vi "Unloading_Queue_States.vi"(7 "QUEUE ST":T2=enum."CLOSE Q", 8 "error in":errorcluster, 11 "Unload St":T1[](array[typedef])) -> (0 "error OUT":errorcluster, 3 "Unload ST":T1)   [LabVIEW 2017]
uses:
  Controls/QUEUE_STATES.ctl
  Controls/Unload_St.ctl
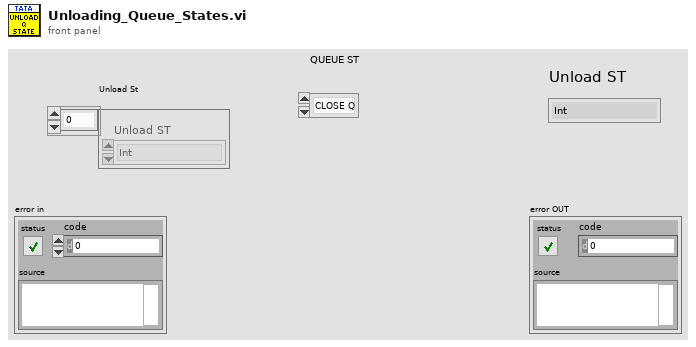
[diagram p1: front panel]
types:
  T1 = typedef "Unload_St.ctl" = enum16{"Int", "Int 2", "Wait", "Cluster_update", "Empty_Bin_Check", "Check_Section_to_Run", "Open_Door", "QR_Scanned", "Close_Door", "Error_Handler", "Stop"}
  T2 = typedef "QUEUE_STATES.ctl" = enum16{"CREATE Q", "EN Q", "DE Q", "CLOSE Q"}
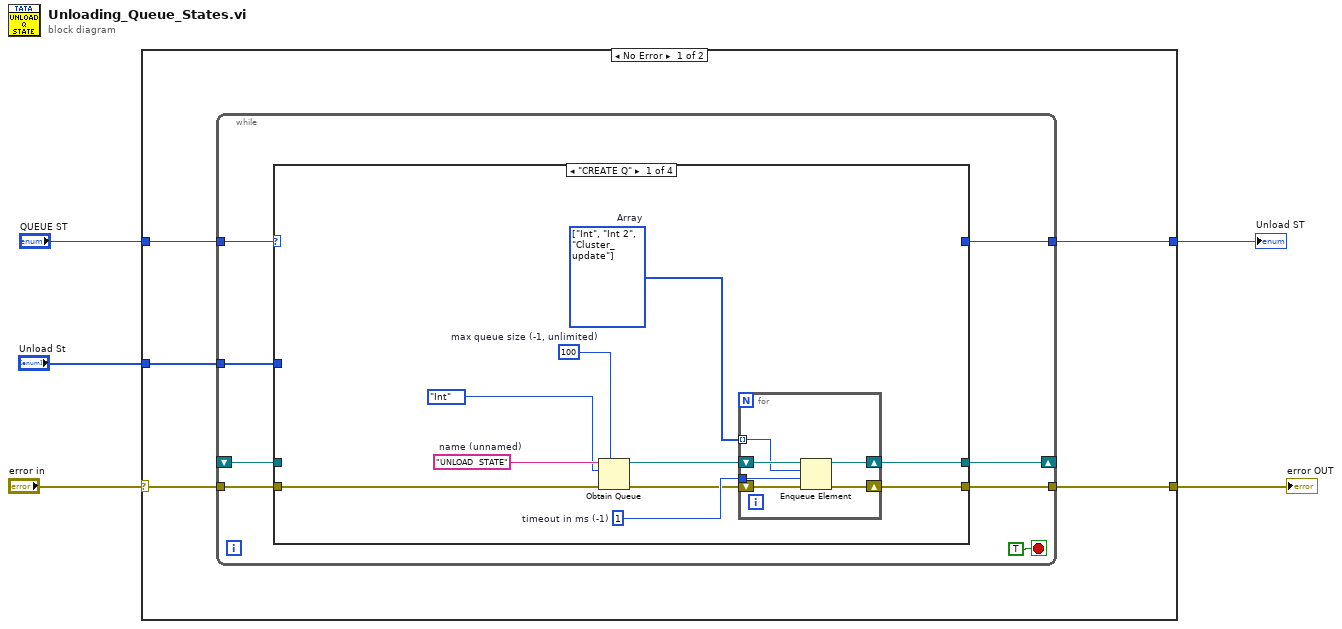
[diagram p0: block diagram]
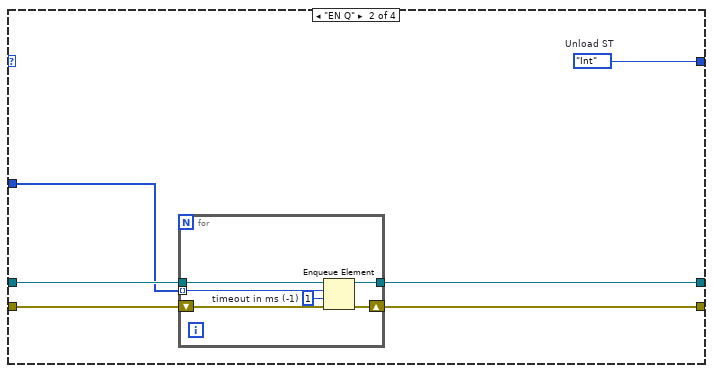
[diagram p2: hidden frame]
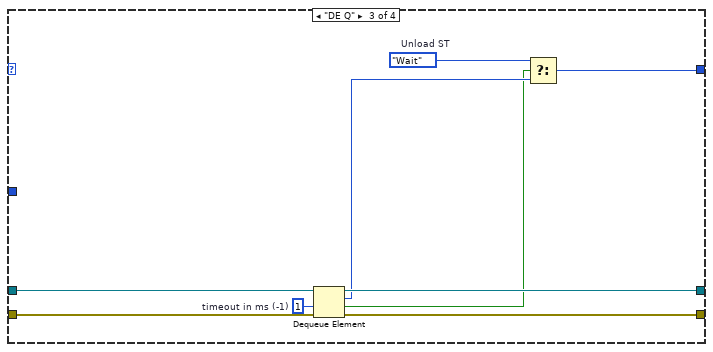
[diagram p3: hidden frame]
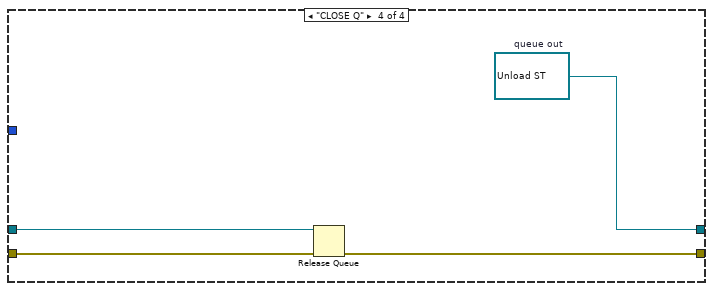
[diagram p4: hidden frame]
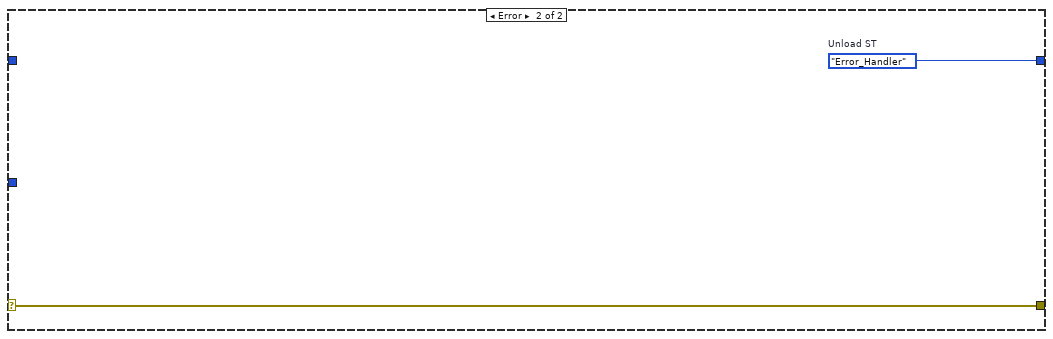
[diagram p5: hidden frame]
diagram:
  n1 = case shown="No Error" "error in" {
    selector: "error in" -> [w10 w61]
    tunnel: [w9 w61] -> w4
    tunnel: [w8 w60] -> w1
    tunnel: "QUEUE ST" -> [w7 _]
    tunnel: "Unload St" -> [w6 _]
    frame No Error {
      n2 = while {
        tunnel: w10 -> [w18]
        tunnel: [w16] -> w9
        tunnel: [w11] -> w8
        tunnel: w7 -> [w15]
        shift-right: [w14] -> _
        shift-left: _ -> [w13]
        tunnel: w6 -> [w12]
        stop <- TRUE stop-if-true
        n3 = case shown="\"CREATE Q\"" w15 {
          tunnel: w18 -> [w28 w40 w55 w59]
          tunnel: [w21 w39 w54 w58] -> w16
          tunnel: [w23 w37 w52 w56] -> w14
          tunnel: w13 -> [_ w38 w53 w57]
          tunnel: w12 -> [_ w36 _ _]
          tunnel: [_ w35 w49 _] -> w11
          frame "CREATE Q" {
            w20 = T1[] [enum."Int", enum."Int 2", enum."Cluster_update"] items=["Int", "Int 2", "Wait", "Cluster_update", "Empty_Bin_Check", "Check_Section_to_Run", "Open_Door", "QR_Scanned", "Close_Door", "Error_Handler", "Stop"]  # Array
            w25 = 1  # timeout in ms (-1)
            w26 = 100  # max queue size (-1, unlimited)
            w27 = "UNLOAD  STATE"  # name (unnamed)
            n4 = Obtain Queue(max queue size (-1, unlimited)=w26, name (unnamed)=w27, element data type=Unload_St."Int" ("Unload ST"), error in (no error)=w28) -> (queue out=w24:refnum<queue>, error out=w22:errorcluster)  [unwired: 1 in, 1 out]
            n5 = for {
              tunnel: w25 -> [w34]
              tunnel: w20 -> [w29] mode=indexing
              shift-right: [w32] -> w23
              shift-left: w24 -> [w33]
              shift-right: [w30] -> w21
              shift-left: w22 -> [w31]
              n6 = Enqueue Element(queue=w33, element=w29, timeout in ms (-1)=w34, error in (no error)=w31) -> (queue out=w32:refnum<queue>, error out=w30:errorcluster)  [unwired: 1 out]
            }
          }
          frame "EN Q" {
            w35 = Unload_St."Int"  # Unload ST
            n7 = for {
              tunnel: w38 -> [w44]
              tunnel: [w43] -> w37
              tunnel: w36 -> [w42] mode=indexing
              shift-right: [w45] -> w39
              shift-left: w40 -> [w46]
              w41 = 1  # timeout in ms (-1)
              n8 = Enqueue Element(queue=w44, element=w42, timeout in ms (-1)=w41, error in (no error)=w46) -> (queue out=w43:refnum<queue>, error out=w45:errorcluster)  [unwired: 1 out]
            }
          }
          frame "DE Q" {
            w47 = Unload_St."Wait"  # Unload ST
            w51 = 1  # timeout in ms (-1)
            n9 = Dequeue Element(queue=w53, timeout in ms (-1)=w51, error in (no error)=w55) -> (queue out=w52:refnum<queue>, element=w50:T1, timed out?=w48:bool, error out=w54:errorcluster)
            n10 = Select(t=w47, s=w48, f=w50) -> (s? t:f=w49:T1)
          }
          frame "CLOSE Q" {
            w56 = refnum<queue> refnum items=["Int", "Int 2", "Wait", "Cluster_update", "Empty_Bin_Check", "Check_Section_to_Run", "Open_Door", "QR_Scanned", "Close_Door", "Error_Handler", "Stop"]  # queue out
            n11 = Release Queue(queue=w57, error in (no error)=w59) -> (error out=w58:errorcluster)  [unwired: 1 in, 2 out]
          }
        }
      }
    }
    frame Error {
      w60 = Unload_St."Error_Handler"  # Unload ST
    }
  }
  "error OUT" <- w4
  "Unload ST" <- w1
